vi "GT_SetCaptureMode.vi"(3 "Mode":u16(ring) items=["Home", "Index", "Probe"], 4 "encoder":i16, 5 "rtn_In":cluster{"rtn":i16, "Func":string}) -> (1 "encoder out":i16, 2 "rtn_Out":cluster{"rtn":i16, "Func":string})   [LabVIEW 2014]
uses:
  VC6/gts.dll
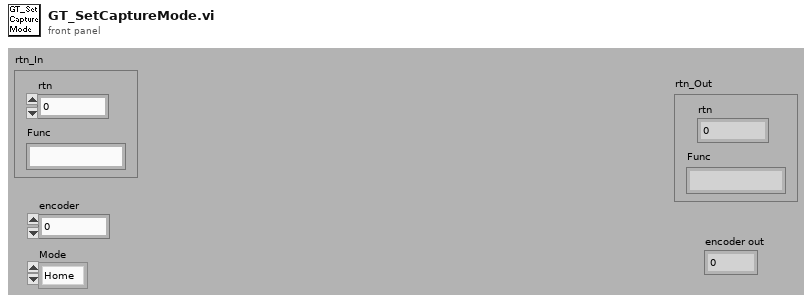
[diagram p1: front panel]
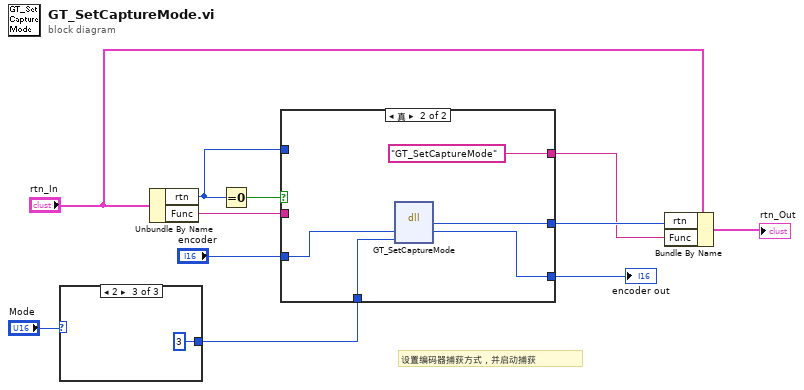
[diagram p0: block diagram]
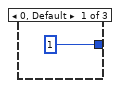
[diagram p2: hidden frame]
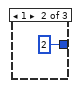
[diagram p3: hidden frame]
diagram:
  # "设置编码器捕获方式，并启动捕获"
  n1 = case shown="2" "Mode" {
    tunnel: [i16 1 ("mode") i16 2 ("mode") i16 3 ("mode")] -> w2
    frame 0, Default {
    }
    frame 1 {
    }
    frame 2 {
    }
  }
  n2 = Unbundle By Name("rtn_In") -> ("rtn"=w6:i16, "Func"=w5:string)
  n3 = Equal To 0?(x=w6) -> (x = 0?=w11:bool)
  n4 = case shown="真" w11 {
    tunnel: [w17 w22] -> w8
    tunnel: [w16 "GT_SetCaptureMode" ("Func")] -> w7
    tunnel: w6 -> [w17 _]
    tunnel: w5 -> [w16 _]
    tunnel: "encoder" -> [w15 w20]
    tunnel: w2 -> [_ w19]
    tunnel: [w15 w18] -> w1
    frame False {
    }
    frame True {
      n5 = dll-call lib="PTH2Fabs DNewGTS AC-800LWin7版源程序-20170926gts85VC6gts.dll" fn="GT_SetCaptureMode"("encoder"=w20, "mode"=w19) -> ("rtn"=w22:i16, "encoder"=w18:i16)  [unwired: 4 in, 2 out]
    }
  }
  "encoder out" <- w1
  n6 = Bundle By Name(cluster="rtn_In", "rtn"=w8, "Func"=w7) -> (→"rtn_Out":cluster{"rtn":i16, "Func":string})
